vi "SpectroMeterRead1.vi"(2 "error IO":errorcluster caption="error in") -> (0 "error IO 2":errorcluster caption="error out")   [LabVIEW 2018]
panel:
  in  "停止":bool
  in  "开始测量":bool
  in  "更改参数":bool
  out "重频":dbl caption="重复频率" format="%.2f"
  out "脉宽":dbl caption="脉冲宽度" format="%.2f"
  out "时间波形":waveform(dbl)(graph)
  # "光   谱"
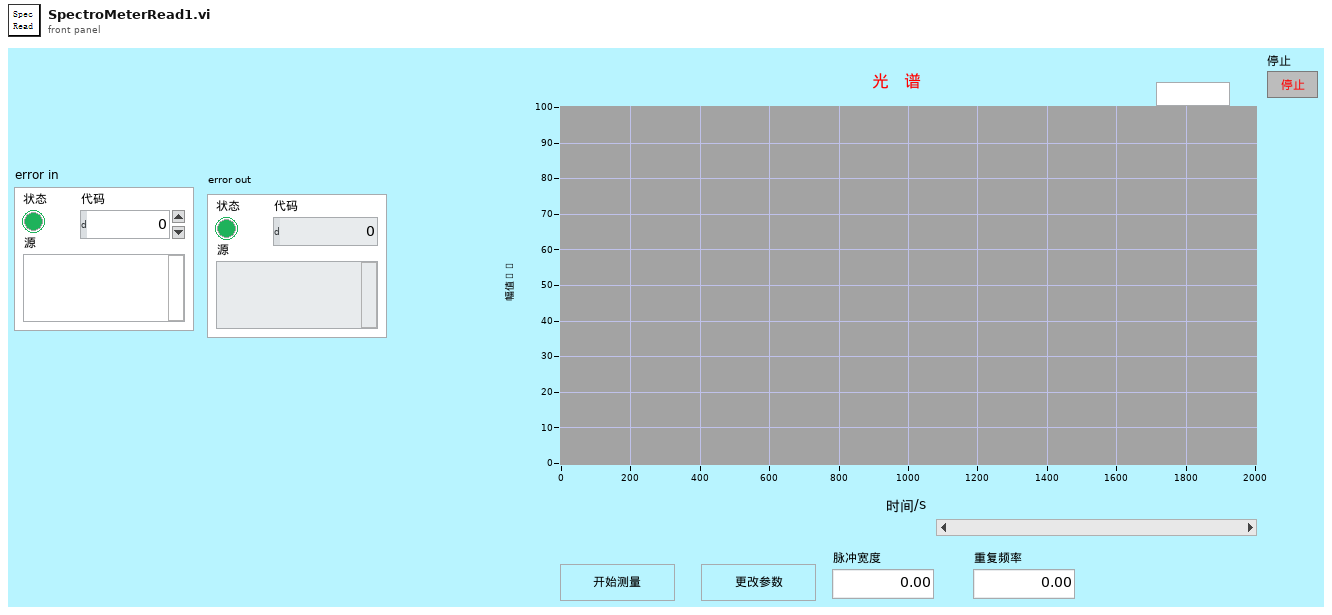
[diagram p1: front panel]
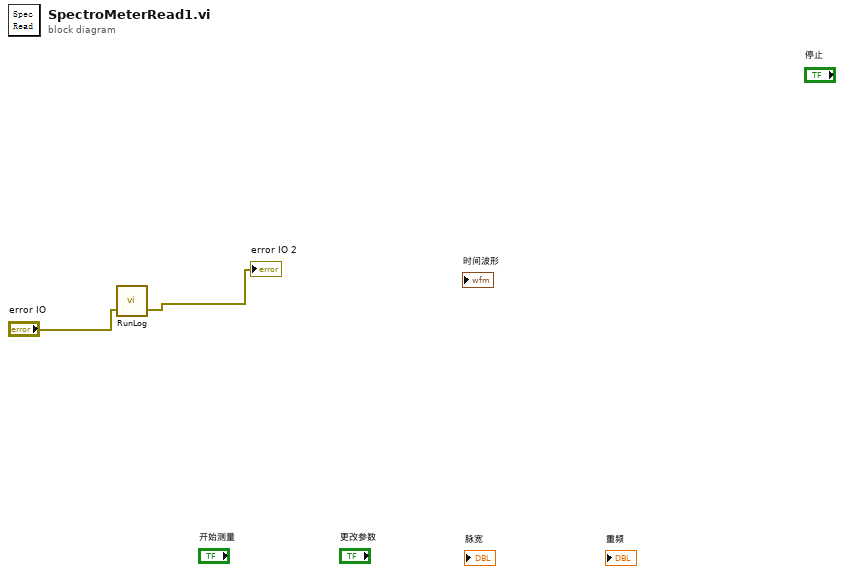
[diagram p0: block diagram]
diagram:
  n1 = call "RunLog.vi"("error in"="error IO") -> ("error out"=→"error IO 2":errorcluster)  [unwired: 2 in]
